vi "Create Timer IRQ.vi"(4 "Callback VI Reference":T1, 8 "error in (no error)":errorcluster, 9 "Interval [us]":u32=1000000, 11 "Timer ID":u8) -> (0 "error out":errorcluster)   [LabVIEW 2021, in "Timer IRQ.lvlib"]
uses:
  <vilib>/myRIO/Instrument Drivers/IRQ/Timer IRQ/Timer IRQ.lvlib
  <vilib>/myRIO/Common/Instrument Driver Framework/myRIO v1.0/IRQ/typedefs/Callback VI Ref.ctl
  <vilib>/myRIO/Instrument Drivers/IRQ/Timer IRQ/vis/myRIO Create Timer IRQ.xnode
  <vilib>/userdefined/High Color/nirio_resource_hc.ctl
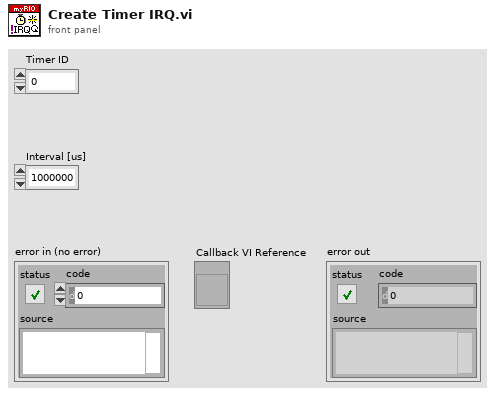
[diagram p1: front panel]
types:
  T1 = typedef "Callback VI Ref.ctl" = refnum<vi>
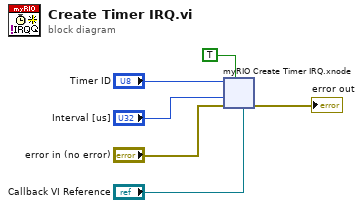
[diagram p0: block diagram]
diagram:
  n1 = xnode "myRIO Create Timer IRQ.xnode"("error in (no error)"="error in (no error)", "Callback VI Reference"="Callback VI Reference", "Allow Overwrite Operation? (F)"=TRUE ("Allow Overwrite? (F)"), "Interval [us]"="Interval [us]", "Timer ID"="Timer ID") -> ("error out"=→"error out":errorcluster)
